vi "Modify array of SCA states.vi"(8 "Current State":T1, 10 "Array of states to process":T1[](array[typedef])) -> (1 "Next State":T1, 3 "Modified Array of states":T1[](array[typedef]))   [LabVIEW 2016]
doc: "Modify Array of States takes the \"Current State\" enum and removes it from the \"Array of States to Processs\" enum array to create the \"Modified Array of States\" enum array which can then be used to properly run the state machine. \n\nThe \"Modified Array of States\" along with the \"Next State\" to process is produced."
uses:
  Beamline sections/Sample Changer A/controls/SCA states.ctl
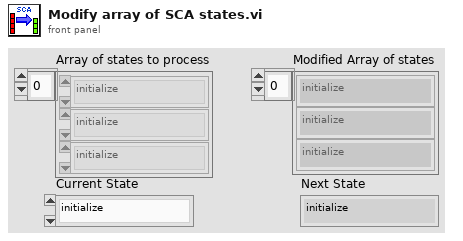
[diagram p1: front panel]
types:
  T1 = typedef "SCA states.ctl" = enum16{"initialize", "wait", "change sample start", "change sample", "check position", "rotate wheel", "sample change complete", "sample rod up", "sample rod down", "retract rod in", "retract rod out", "insert rod in", "insert rod out", "wheel GV open", "wheel GV close", "vent source", "pump source", "shutdown"}
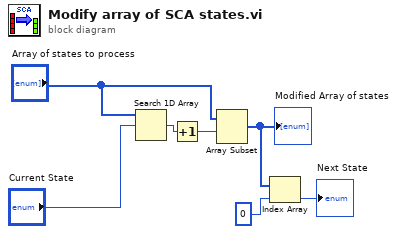
[diagram p0: block diagram]
diagram:
  n1 = Search 1D Array(1D array="Array of states to process", element="Current State") -> (index of element=w6:i32)  [unwired: 1 in]
  n2 = Increment(x=w6) -> (x+1=w7:i32)
  n3 = Array Subset(array="Array of states to process", index=w7) -> (w1:T1[])  [unwired: 1 in]
  "Modified Array of states" <- w1
  n4 = Index Array(array=w1, index=0) -> (element=→"Next State":T1)
